vi "Test Map to Array.vi"() -> ()   [LabVIEW 2020]
uses:
  2266703d-64b8-42de-a1e2-478899a8b022.vi
  cc5ec10c-74fc-454e-b6f1-bdc72e1dc85f.vi
  2266703d-64b8-42de-a1e2-478899a8b022.vi/b0178052-0c48-4c9a-874f-40b592e34ac5.vi
  <vilib>/addons/_JKI Toolkits/Caraya/Caraya.lvlibp/1abvi3w/vi.lib/addons/_JKI Toolkits/Caraya/classes/Assert/Assert Equal Value and Type_Variant.vi
  <vilib>/addons/_JKI Toolkits/Caraya/Caraya.lvlibp/1abvi3w/vi.lib/addons/_JKI Toolkits/Caraya/classes/Test/Test.lvclass
  <vilib>/addons/_JKI Toolkits/Caraya/Caraya.lvlibp/1abvi3w/vi.lib/addons/_JKI Toolkits/Caraya/classes/Assert/Assert.lvclass
panel:
  out "error out":errorcluster
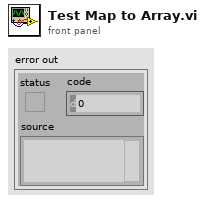
[diagram p1: front panel]
types:
  T1 = cluster{"Name":i32, "value":cluster{"bool":bool, "string":string}}[]
  T2 = cluster{"key type":i32, "value type":cluster{"bool":bool, "string":string}}[]
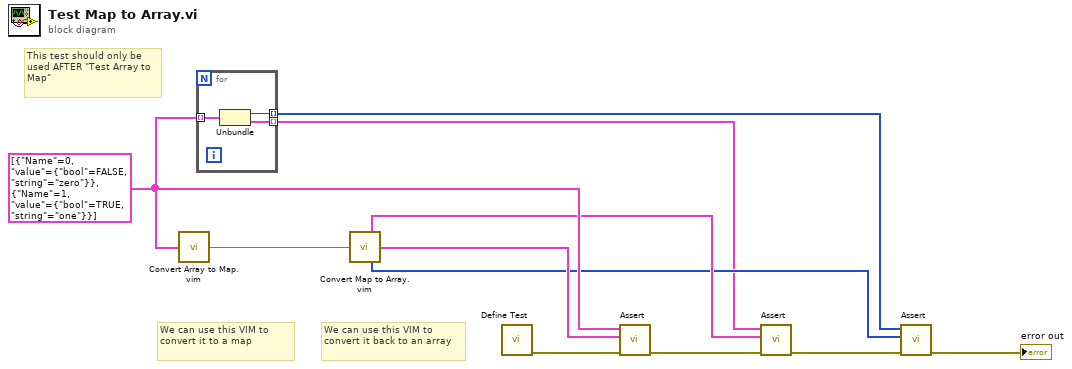
[diagram p0: block diagram]
diagram:
  w8 = T1 [{"Name"=0, "value"={"bool"=FALSE, "string"="zero"}}, {"Name"=1, "value"={"bool"=TRUE, "string"="one"}}] ("Array")
  # "We can use this VIM to convert it back to an array"
  # "This test should only be used AFTER \"Test Array to Map\""
  # "We can use this VIM to convert it to a map"
  n1 = call "Convert Array to Map.vim"("array"=w8) -> ("map"=w10:map{i32, cluster{"bool":bool, "string":string}})  [unwired: 6 in]
  n2 = for {
    tunnel: w8 -> [w14] mode=indexing
    tunnel: [w13] -> w1 mode=indexing
    tunnel: [w12] -> w2 mode=indexing
    n3 = Unbundle(w14) -> ("Name"=w13:i32, "value"=w12:cluster{"bool":bool, "string":string})
  }
  n4 = call "Convert Map to Array.vim"("map"=w10) -> ("keys"=w3:i32[], "array"=w4:T2, "values"=w7:cluster{"bool":bool, "string":string}[])  [unwired: 12 in]
  n5 = call <vilib>:"Define Test.vi"() -> ("error out"=w11:errorcluster)  [unwired: 11 in]
  n6 = call-poly <vilib>:"Assert.vi"("error in (no error)"=w11, "Y"=w4, "X"=w8) -> ("error out"=w9:errorcluster)  [unwired: 8 in]
  n7 = call-poly <vilib>:"Assert.vi"("error in (no error)"=w9, "Y"=w7, "X"=w2) -> ("error out"=w6:errorcluster)  [unwired: 8 in]
  n8 = call-poly <vilib>:"Assert.vi"("error in (no error)"=w6, "Y"=w3, "X"=w1) -> ("error out"=→"error out":errorcluster)  [unwired: 8 in]
